vi "grow tree.vi"(8 "variant in":variant, 10 "tokens":T1[](array[typedef]), 11 "String":string) -> (0 "variant out":variant, 2 "remaining tokens":T1[](array[typedef]))   [LabVIEW 2013]
uses:
  json token.ctl
  json node type.ctl
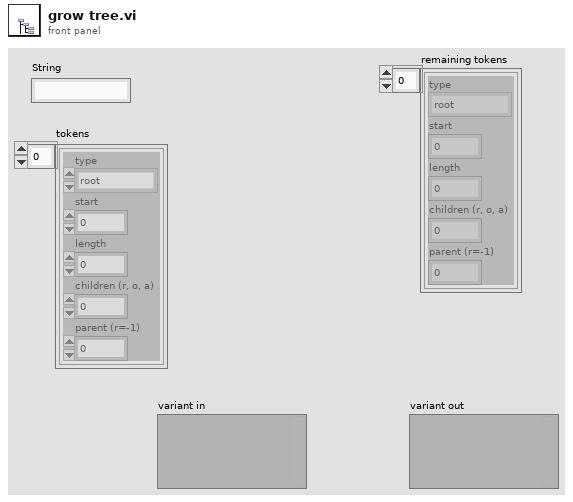
[diagram p1: front panel]
types:
  T1 = typedef "json token.ctl" = cluster{"type":T2, "start":i32, "length":i32, "children (r, o, a)":u16, "parent (r=-1)":i32}
  T2 = typedef "json node type.ctl" = enum16{"root", "object", "array", "number", "string value", "string key", "true", "false", "null"}
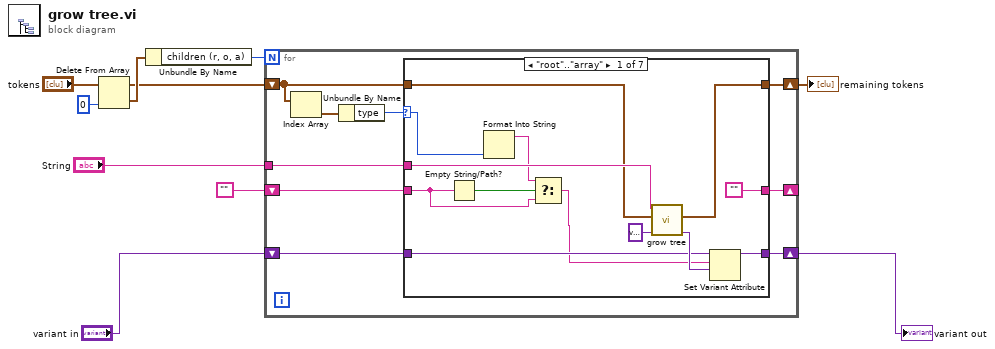
[diagram p0: block diagram]
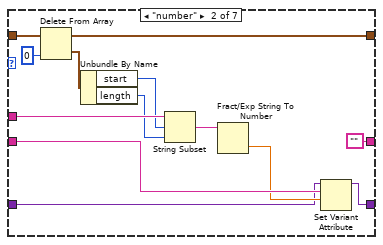
[diagram p2: hidden frame]
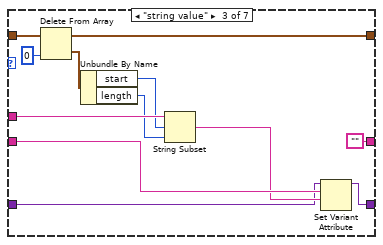
[diagram p3: hidden frame]
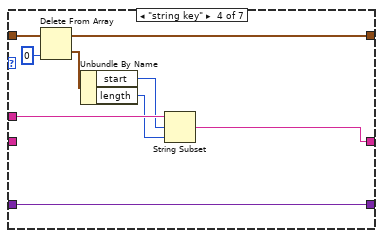
[diagram p4: hidden frame]
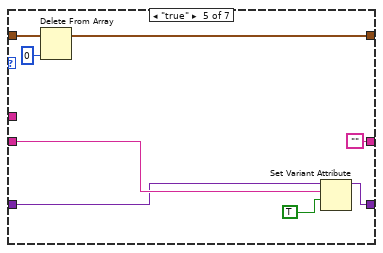
[diagram p5: hidden frame]
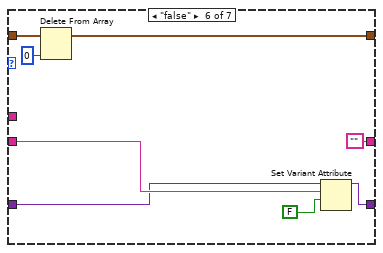
[diagram p6: hidden frame]
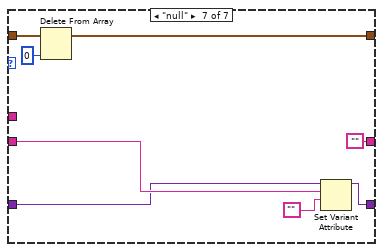
[diagram p7: hidden frame]
diagram:
  n1 = Delete From Array(array="tokens", index=0) -> (deleted portion=w8:T1, array with subset deleted=w7:T1[])  [unwired: 1 in]
  n2 = Unbundle By Name(w8) -> ("children (r, o, a)"=w6:u16)
  n3 = for {
    N: w6 -> [_]
    tunnel: "String" -> [w17]
    shift-right: [w14] -> _
    shift-left: "" -> [w18]
    shift-right: [w15] -> w4
    shift-left: w7 -> [w16]
    shift-right: [w12] -> w1
    shift-left: "variant in" -> [w11]
    n4 = Index Array(array=w16) -> (element=w13:T1)  [unwired: 1 in]
    n5 = Unbundle By Name(w13) -> ("type"=w19:T2)
    n6 = case shown="\"root\"..\"array\"" w19 {
      selector: w19 -> [w25 _ _ _ _ _ _]
      tunnel: w18 -> [w27 w36 w49 _ w70 w78 w86]
      tunnel: w17 -> [w32 w40 w52 w62 _ _ _]
      tunnel: w16 -> [w31 w44 w56 w66 w73 w81 w89]
      tunnel: [w30 w43 w55 w65 w72 w80 w88] -> w15
      tunnel: ["" "" "" w59 "" "" ""] -> w14
      tunnel: [w23 w34 w47 w58 w68 w76 w84] -> w12
      tunnel: w11 -> [w22 w33 w46 w58 w67 w75 w83]
      frame "root".."array" {
        n7 = Empty String/Path?(string/path=w27) -> (empty?=w28:bool)
        n8 = Format Into String(w25) -> (resulting string=w26:string)  [unwired: 3 in, 1 out]
        n9 = Select(t=w26, s=w28, f=w27) -> (s? t:f=w20:string)
        n10 = call "grow tree.vi"("variant in"=variant, "tokens"=w31, "String"=w32) -> ("variant out"=w24:variant, "remaining tokens"=w30:T1[])  [unwired: 7 in]
        n11 = Set Variant Attribute(Variant=w22, name=w20, value=w24) -> (Variant out=w23:variant)  [unwired: 1 in, 2 out]
      }
      frame "number" {
        n12 = Delete From Array(array=w44, index=0) -> (deleted portion=w41:T1, array with subset deleted=w43:T1[])  [unwired: 1 in]
        n13 = Unbundle By Name(w41) -> ("start"=w39:i32, "length"=w38:i32)
        n14 = String Subset(string=w40, offset (0)=w39, length (rest)=w38) -> (substring=w37:string)
        n15 = Fract/Exp String To Number(string=w37) -> (number=w35:dbl)  [unwired: 3 in, 1 out]
        n16 = Set Variant Attribute(Variant=w33, name=w36, value=w35) -> (Variant out=w34:variant)  [unwired: 1 in, 2 out]
      }
      frame "string value" {
        n17 = Delete From Array(array=w56, index=0) -> (deleted portion=w53:T1, array with subset deleted=w55:T1[])  [unwired: 1 in]
        n18 = Unbundle By Name(w53) -> ("start"=w51:i32, "length"=w50:i32)
        n19 = String Subset(string=w52, offset (0)=w51, length (rest)=w50) -> (substring=w48:string)
        n20 = Set Variant Attribute(Variant=w46, name=w49, value=w48) -> (Variant out=w47:variant)  [unwired: 1 in, 2 out]
      }
      frame "string key" {
        n21 = Delete From Array(array=w66, index=0) -> (deleted portion=w63:T1, array with subset deleted=w65:T1[])  [unwired: 1 in]
        n22 = Unbundle By Name(w63) -> ("start"=w61:i32, "length"=w60:i32)
        n23 = String Subset(string=w62, offset (0)=w61, length (rest)=w60) -> (substring=w59:string)
      }
      frame "true" {
        n24 = Delete From Array(array=w73, index=0) -> (array with subset deleted=w72:T1[])  [unwired: 1 in, 1 out]
        n25 = Set Variant Attribute(Variant=w67, name=w70, value=TRUE) -> (Variant out=w68:variant)  [unwired: 1 in, 2 out]
      }
      frame "false" {
        n26 = Delete From Array(array=w81, index=0) -> (array with subset deleted=w80:T1[])  [unwired: 1 in, 1 out]
        n27 = Set Variant Attribute(Variant=w75, name=w78, value=FALSE) -> (Variant out=w76:variant)  [unwired: 1 in, 2 out]
      }
      frame "null" {
        n28 = Delete From Array(array=w89, index=0) -> (array with subset deleted=w88:T1[])  [unwired: 1 in, 1 out]
        n29 = Set Variant Attribute(Variant=w83, name=w86, value="") -> (Variant out=w84:variant)  [unwired: 1 in, 2 out]
      }
    }
  }
  "variant out" <- w1
  "remaining tokens" <- w4
